vi "Convert V to g.vi"(10 "channel":i32, 11 "Accelerometer Voltage (V)":fxp<+/-,24,4>) -> (3 "Acceleration (g)":sgl)   [LabVIEW 2017]
doc: "Convert accelerometer voltage (V) to acceleration (g)."
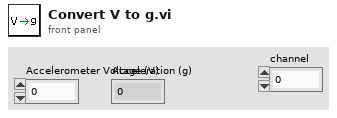
[diagram p1: front panel]
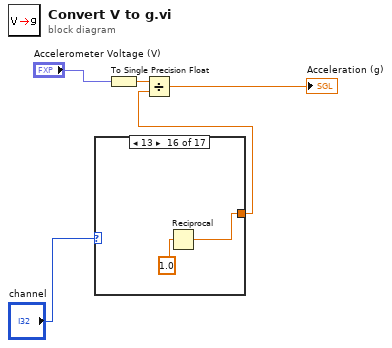
[diagram p0: block diagram]
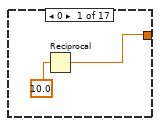
[diagram p2: hidden frame]
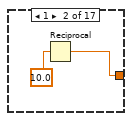
[diagram p3: hidden frame]
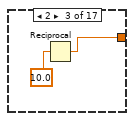
[diagram p4: hidden frame]
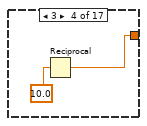
[diagram p5: hidden frame]
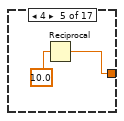
[diagram p6: hidden frame]
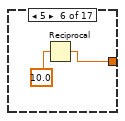
[diagram p7: hidden frame]
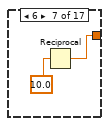
[diagram p8: hidden frame]
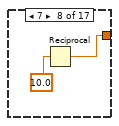
[diagram p9: hidden frame]
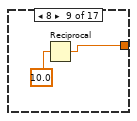
[diagram p10: hidden frame]
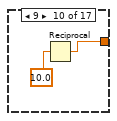
[diagram p11: hidden frame]
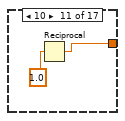
[diagram p12: hidden frame]
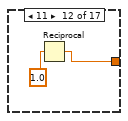
[diagram p13: hidden frame]
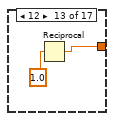
[diagram p14: hidden frame]
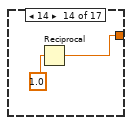
[diagram p15: hidden frame]
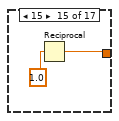
[diagram p16: hidden frame]
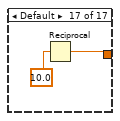
[diagram p17: hidden frame]
diagram:
  n1 = case shown="13" "channel" {
    tunnel: [w7 w8 w10 w12 w14 w16 w18 w20 w22 w24 w26 w28 w30 w32 w34 w36 w38] -> w2
    frame 0 {
      n2 = Reciprocal(x=sgl 10.0 ("y")) -> (1/x=w7:sgl)
    }
    frame 1 {
      n3 = Reciprocal(x=sgl 10.0 ("y")) -> (1/x=w8:sgl)
    }
    frame 2 {
      n4 = Reciprocal(x=sgl 10.0 ("y")) -> (1/x=w10:sgl)
    }
    frame 3 {
      n5 = Reciprocal(x=sgl 10.0 ("y")) -> (1/x=w12:sgl)
    }
    frame 4 {
      n6 = Reciprocal(x=sgl 10.0 ("y")) -> (1/x=w14:sgl)
    }
    frame 5 {
      n7 = Reciprocal(x=sgl 10.0 ("y")) -> (1/x=w16:sgl)
    }
    frame 6 {
      n8 = Reciprocal(x=sgl 10.0 ("y")) -> (1/x=w18:sgl)
    }
    frame 7 {
      n9 = Reciprocal(x=sgl 10.0 ("y")) -> (1/x=w20:sgl)
    }
    frame 8 {
      n10 = Reciprocal(x=sgl 10.0 ("y")) -> (1/x=w22:sgl)
    }
    frame 9 {
      n11 = Reciprocal(x=sgl 10.0 ("y")) -> (1/x=w24:sgl)
    }
    frame 10 {
      n12 = Reciprocal(x=sgl 1.0 ("y")) -> (1/x=w26:sgl)
    }
    frame 11 {
      n13 = Reciprocal(x=sgl 1.0 ("y")) -> (1/x=w28:sgl)
    }
    frame 12 {
      n14 = Reciprocal(x=sgl 1.0 ("y")) -> (1/x=w30:sgl)
    }
    frame 14 {
      n15 = Reciprocal(x=sgl 1.0 ("y")) -> (1/x=w32:sgl)
    }
    frame 15 {
      n16 = Reciprocal(x=sgl 1.0 ("y")) -> (1/x=w34:sgl)
    }
    frame 13 {
      n17 = Reciprocal(x=sgl 1.0 ("y")) -> (1/x=w36:sgl)
    }
    frame Default {
      n18 = Reciprocal(x=sgl 10.0 ("y")) -> (1/x=w38:sgl)
    }
  }
  n19 = To Single Precision Float(number="Accelerometer Voltage (V)") -> (single precision float=w3:sgl)
  n20 = Divide(x=w3, y=w2) -> (x/y=→"Acceleration (g)":sgl)
